vi "FindShootingInvaders.vi"(1 "MainCluster_IN":T11) -> (0 "MainCluster_OUT":T11)   [LabVIEW 2022 SP3]
uses:
  InitCluster.ctl
  CharacterCluster.ctl
  <vilib>/picture/picture.llb/imagedata.ctl
  ShotInitCluster.ctl
  <vilib>/Utility/miscctls.llb/LVPositionTypeDef.ctl
  <vilib>/Utility/miscctls.llb/LVBoundsTypeDef.ctl
  ShotCluster.ctl
  move_dir_ud.ctl
  InvaderPositionArray.ctl
  move_dir_lr.ctl
  <vilib>/numeric/Random Number (Range) U64.vi
  <vilib>/numeric/sub_Random U32.vi
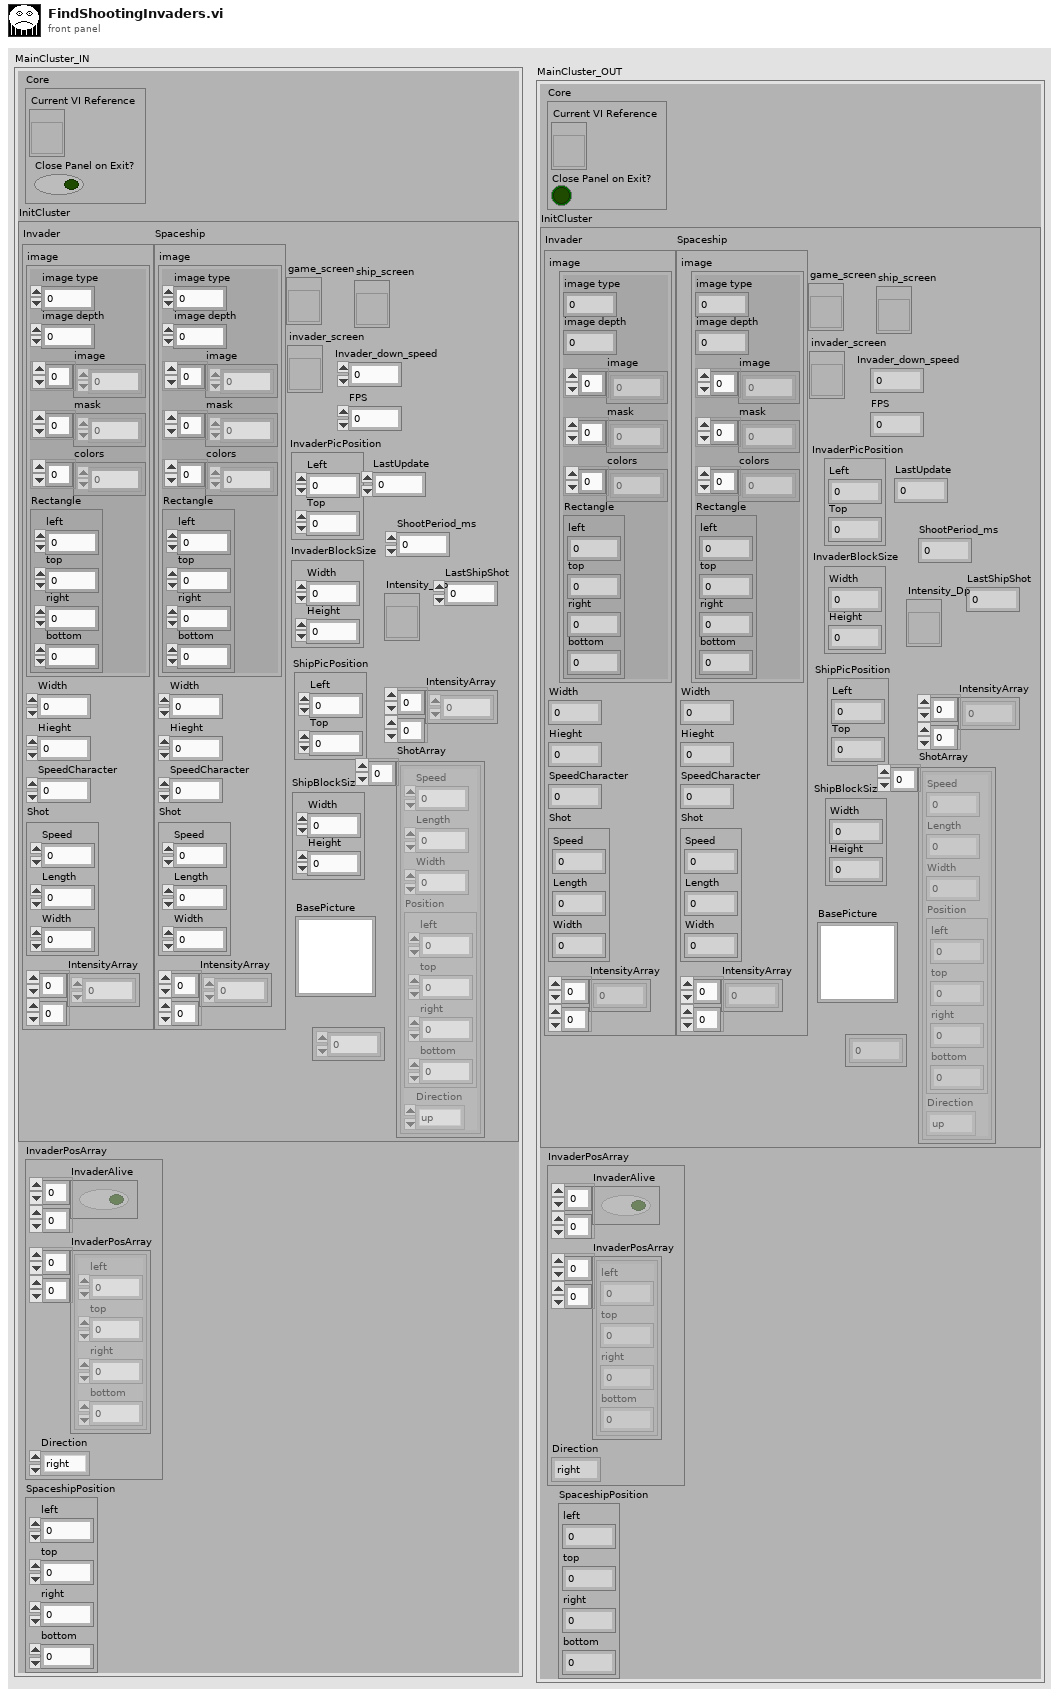
[diagram p1: front panel]
types:
  T1 = typedef "InitCluster.ctl" = cluster{"Invader":T2, "Spaceship":T2, "game_screen":refnum<vi>, "BasePicture":picture, "invader_screen":refnum<vi>, "InvaderPicPosition":T5, "Invader_down_speed":i16, "FPS":u16, "InvaderBlockSize":T6, "ship_screen":refnum<vi>, "ShipBlockSize":T6, "ShipPicPosition":T5, "LastUpdate":u32, "Intensity_Dp":refnum<vi>, "IntensityArray":u8[][], "ShotArray":T7[], "InvaderShotTimeArray":u32[], "ShootPeriod_ms":i32, "LastShipShot":u32}
  T2 = typedef "CharacterCluster.ctl" = cluster{"image":T3, "Width":u32, "Hieght":u32, "SpeedCharacter":u32, "Shot":T4, "IntensityArray":u8[][]}
  T3 = typedef "imagedata.ctl" = cluster{"image type":i32, "image depth":i32, "image":u8[], "mask":u8[], "colors":u32[], "Rectangle":cluster{"left":i16, "top":i16, "right":i16, "bottom":i16}}
  T4 = typedef "ShotInitCluster.ctl" = cluster{"Speed":u32, "Length":u32, "Width":u32}
  T5 = typedef "LVPositionTypeDef.ctl" = cluster{"Left":i32, "Top":i32}
  T6 = typedef "LVBoundsTypeDef.ctl" = cluster{"Width":u32, "Height":u32}
  T7 = typedef "ShotCluster.ctl" = cluster{"Speed":u32, "Length":u32, "Width":u32, "Position":cluster{"left":i16, "top":i16, "right":i16, "bottom":i16}, "Direction":T8}
  T8 = typedef "move_dir_ud.ctl" = enum16{"up", "down"}
  T9 = typedef "InvaderPositionArray.ctl" = cluster{"InvaderAlive":bool[][], "InvaderPosArray":cluster{"left":i16, "top":i16, "right":i16, "bottom":i16}[][], "Direction":T10}
  T10 = typedef "move_dir_lr.ctl" = enum16{"right", "left"}
  T11 = cluster{"Core":cluster{"Current VI Reference":refnum<vi>, "Close Panel on Exit?":bool}, "InitCluster":T1, "InvaderPosArray":T9, "SpaceshipPosition":cluster{"left":i16, "top":i16, "right":i16, "bottom":i16}}
  T12 = cluster{"left":i16, "top":i16, "right":i16, "bottom":i16}[][]
  T13 = cluster{"left":i16, "top":i16, "right":i16, "bottom":i16}
  T14 = cluster{"left":i16, "top":i16, "right":i16, "bottom":i16}[]
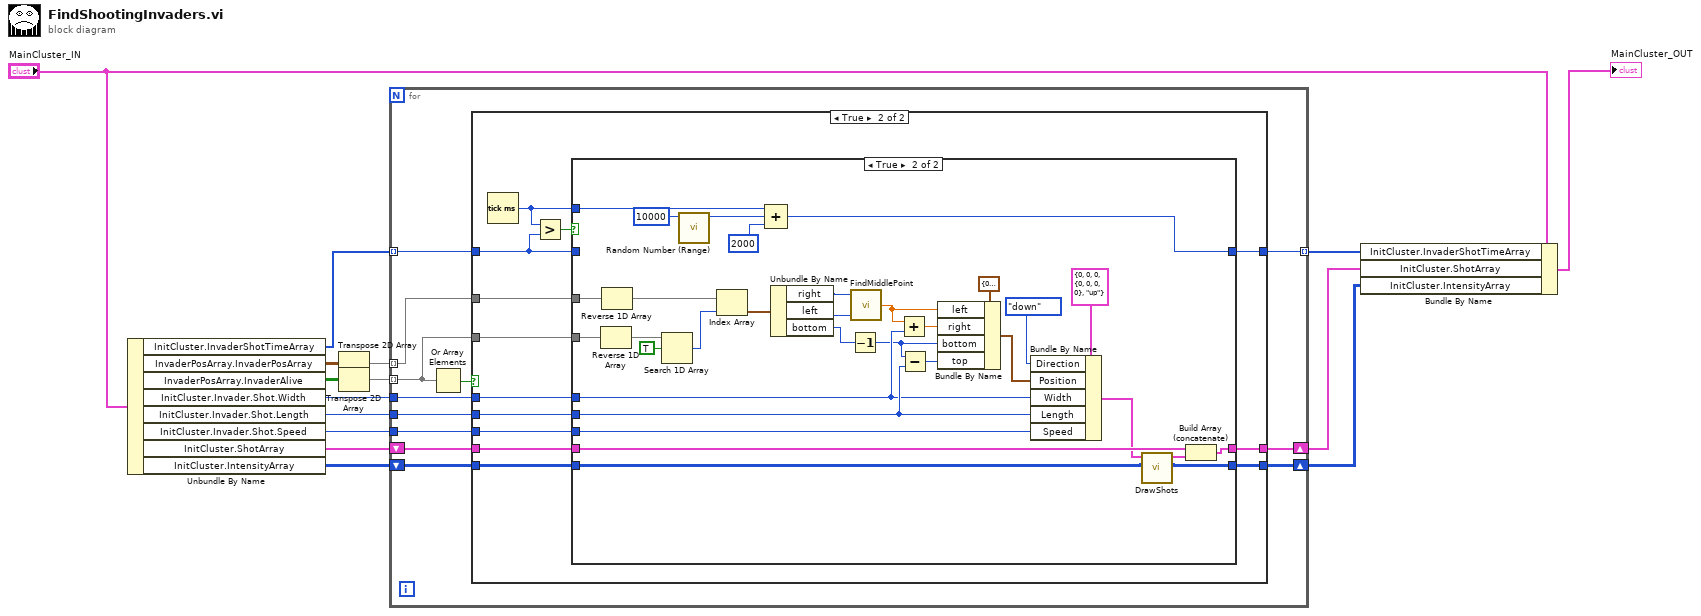
[diagram p0: block diagram]
diagram:
  n1 = Unbundle By Name("MainCluster_IN") -> ("InitCluster.InvaderShotTimeArray"=w11:u32[], "InvaderPosArray.InvaderPosArray"=w13:T12, "InvaderPosArray.InvaderAlive"=w15:bool[][], "InitCluster.Invader.Shot.Width"=w7:u32, "InitCluster.Invader.Shot.Length"=w6:u32, "InitCluster.Invader.Shot.Speed"=w5:u32, "InitCluster.ShotArray"=w4:T7[], "InitCluster.IntensityArray"=w2:u8[][])
  n2 = Transpose 2D Array(2D array=w13) -> (transposed array=w14:T12)
  n3 = Transpose 2D Array(2D array=w15) -> (transposed array=w12:bool[][])
  n4 = for {
    tunnel: w12 -> [w24] mode=indexing
    tunnel: w11 -> [w27] mode=indexing
    tunnel: w14 -> [w25] mode=indexing
    tunnel: [w23] -> w8 mode=indexing
    tunnel: w7 -> [w22]
    tunnel: w6 -> [w21]
    tunnel: w5 -> [w20]
    shift-right: [w18] -> w3
    shift-left: w4 -> [w19]
    shift-right: [w16] -> w1
    shift-left: w2 -> [w17]
    n5 = Or Array Elements(Boolean array=w24) -> (logical OR=w26:bool)
    n6 = case shown="True" w26 {
      tunnel: w27 -> [w30 w40]
      tunnel: w25 -> [_ w42]
      tunnel: w24 -> [_ w43]
      tunnel: [w30 w39] -> w23
      tunnel: w22 -> [_ w37]
      tunnel: w21 -> [_ w36]
      tunnel: w20 -> [_ w35]
      tunnel: w19 -> [w29 w34]
      tunnel: [w29 w33] -> w18
      tunnel: w17 -> [w28 w32]
      tunnel: [w28 w31] -> w16
      frame False {
      }
      frame True {
        n7 = Tick Count (ms)() -> (millisecond timer value=w38:u32)
        n8 = Greater?(x=w38, y=w40) -> (0:w41:bool)
        n9 = case shown="True" w41 {
          tunnel: w43 -> [_ w77]
          tunnel: w42 -> [_ w75]
          tunnel: w40 -> [w46 _]
          tunnel: [w46 w68] -> w39
          tunnel: w38 -> [_ w70]
          tunnel: w37 -> [_ w54]
          tunnel: w36 -> [_ w59]
          tunnel: w35 -> [_ w60]
          tunnel: w34 -> [w45 w56]
          tunnel: [w45 w55] -> w33
          tunnel: w32 -> [w44 w48]
          tunnel: [w44 w47] -> w31
          frame False {
          }
          frame True {
            n10 = Reverse 1D Array(array=w77) -> (reversed array=w78:bool[])
            n11 = Reverse 1D Array(array=w75) -> (reversed array=w74:T14)
            n12 = Search 1D Array(1D array=w78, element=TRUE) -> (index of element=w73:i32)  [unwired: 1 in]
            n13 = call-poly <vilib>:"Random Number (Range).vi"("upper bound (100)"=u64 10000) -> ("number"=w71:u64)  [unwired: 10 in]
            n14 = Index Array(array=w74, index=w73) -> (element=w66:T13)
            n15 = Compound Arithmetic op=ADD(w70, w71, u64 2000 ("value")) -> (w68:u64)
            n16 = Unbundle By Name(w66) -> ("right"=w65:i16, "left"=w64:i16, "bottom"=w52:i16)
            n17 = Decrement(x=w52) -> (x-1=w51:i16)
            n18 = call "FindMiddlePoint.vi"("left"=w64, "right"=w65) -> ("middle"=w63:dbl)  [unwired: 3 in]
            n19 = Add(x=w63, y=w54) -> (x+y=w62:dbl)
            n20 = Subtract(x=w51, y=w59) -> (x-y=w53:u32)
            n21 = Bundle By Name(cluster=T13 {"left"=0, "top"=0, "right"=0, "bottom"=0} ("Rectangle"), "left"=w63, "right"=w62, "bottom"=w51, "top"=w53) -> (w58:T13)
            n22 = Bundle By Name(cluster=T7 {"Speed"=0, "Length"=0, "Width"=0, "Position"={"left"=0, "top"=0, "right"=0, "bottom"=0}, "Direction"=enum."up"} ("Shot"), "Direction"=move_dir_ud."down", "Position"=w58, "Width"=w54, "Length"=w59, "Speed"=w60) -> (w50:T7)
            n23 = call "DrawShots.vi"("IntensityArray_IN"=w48, "Shot"=w50) -> ("IntensityArray_OUT"=w47:u8[][], "Shot_OUT"=w49:T7)  [unwired: 8 in]
            n24 = Build Array (concatenate)(w56, w49) -> (w55:T7[])
          }
        }
      }
    }
  }
  n25 = Bundle By Name(cluster="MainCluster_IN", "InitCluster.InvaderShotTimeArray"=w8, "InitCluster.ShotArray"=w3, "InitCluster.IntensityArray"=w1) -> (→"MainCluster_OUT":T11)
